vi "main.vi"() -> ()   [LabVIEW 2013]
doc: "Use this template to parse data you acquired from an instrument and write the data to a file.\nNote: LabVIEW enables automatic error handling by default for VIs you create from this template."
uses:
  Instance           1 22Saved   Instr_Read.vit .vi
  <vilib>/express/express shared/transition.llb/Dynamic To Waveform Array.vi
  <vilib>/Utility/file.llb/Write To Spreadsheet File (DBL).vi
  <vilib>/express/express signal manip/GetorSetDDTAttributes/Get DDT Attributes/Get DDT Properties.xnode
panel:
  out "Timestamp":timestamp
  in  "Pressão":dbl
  in  "Vazão":dbl
  out "P1 3":dbl(knob) scale=0.0..10.0
  out "P1 2":dbl(knob) scale=0.0..10.0
  out "P1":dbl(knob) scale=0.0..10.0 scale format="%#_2g"
  out "EMCA":cluster{dbl, dbl}(slide) scale=0.0..100.0 scale format="%#.2f %%"
  out "Água":dbl(slide) scale=0.0..100.0 scale format="%#.2f %%"
  out "ÁGUA\n              DE \nDESLOCAMENTO":dbl(slide) scale=0.0..100.0 scale format="%#.2f %%"
  in  "ON_OFF_Buttom":bool
  in  "Tab Control":enum32{"Entrada", "Aquisição", "Gráficos"}(tab)
  in  "Viscosidade (µ)":dbl=0.1
  in  "Comprimento (L)":dbl=4.0
  in  "Area (A)":dbl=2.0
  in  "Record_Buttom":bool
  in  "Arquivo de Aquisição":path
  in  "Taxa de Aquisição":dbl=1.0
  in  "Taxa de Atualização":dbl=10.0
  out "Waveform Graph 3":dynamicdata(graph)
  out "Waveform Graph 2":dynamicdata(graph)
  out "Waveform Graph 1":dynamicdata(graph)
  # "Bomba"
  # "Core Holder"
  # "On Windows/Linux, consider using the Instrument Driver Finder (Help>>Find Instrument Drivers) to search for an instrument driver for your instrument."
  # "m2"
  # "m"
  # "Pa.s"
  # "S/s"
  # "S/s"
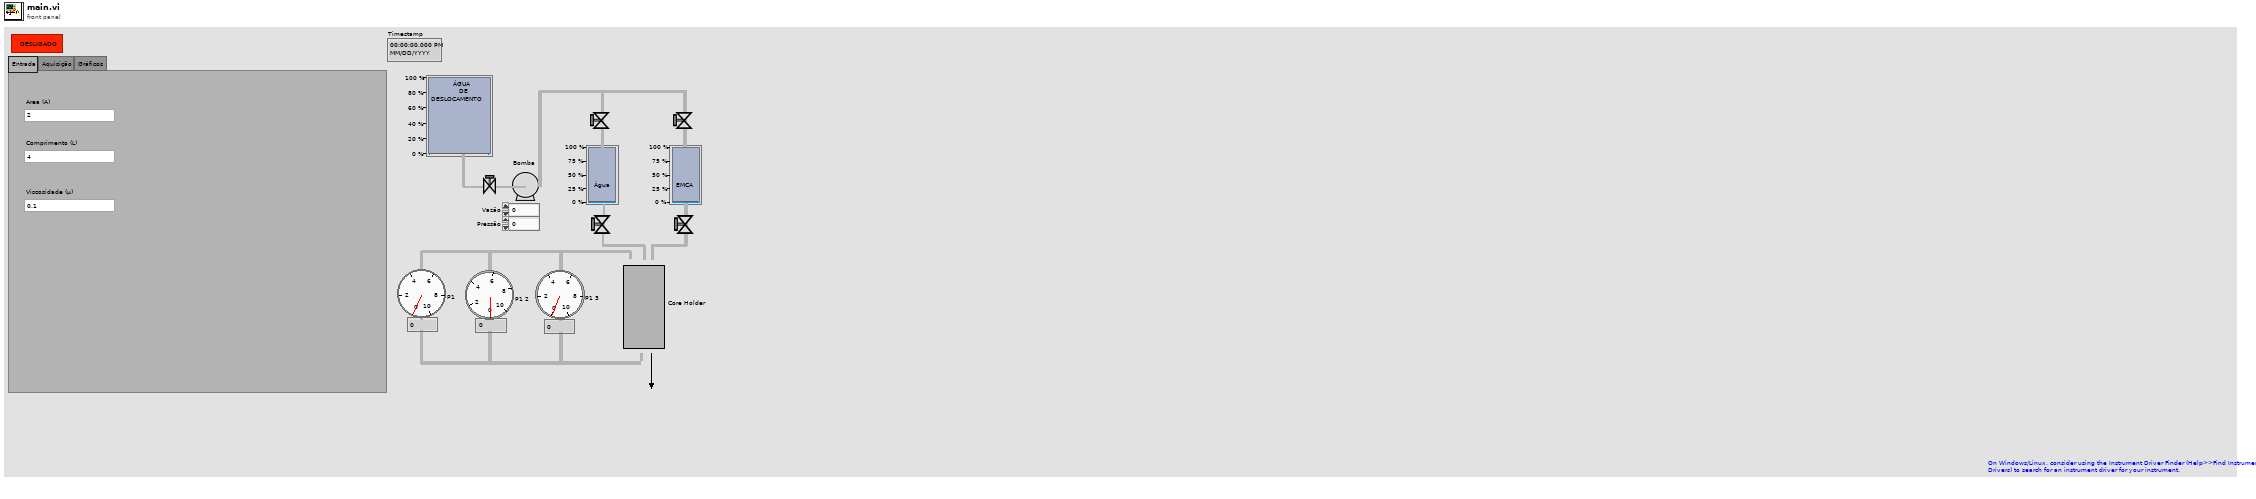
[diagram p1: front panel]
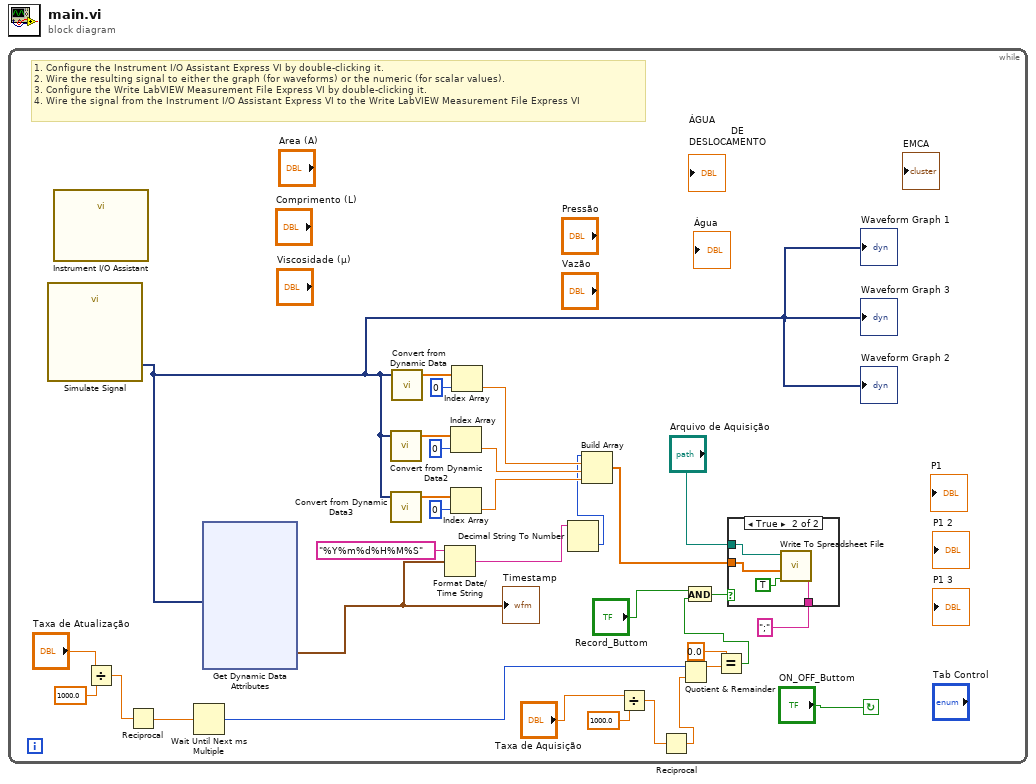
[diagram p0: block diagram]
diagram:
  n1 = while {
    stop <- "ON_OFF_Buttom" continue-if-true
    # "1. Configure the Instrument I/O Assistant Express VI by double-clicking it.\n2. Wire the resulting signal to either the graph (for waveforms) or the numeric (for scalar values).\n3. Configure the Write LabVIEW Measurement File Express VI by double-clicking it.\n4. Wire the signal from the Instrument I/O Assistant Express VI to the Write LabVIEW Measurement File Express VI"
    n2 = call "Simulate Signal"() -> ("Sine"=w9:dynamicdata)  [unwired: 14 in, 1 out]
    "Waveform Graph 3" <- w9
    "Waveform Graph 2" <- w9
    "Waveform Graph 1" <- w9
    n3 = call "Instrument I/O Assistant"() -> ()  [unwired: 12 in]
    n4 = Divide(x="Taxa de Atualização", y=1000.0) -> (x/y=w27:dbl)
    n5 = Reciprocal(x=w27) -> (1/x=w28:dbl)
    n6 = Wait Until Next ms Multiple(millisecond multiple=w28) -> (millisecond timer value=w29:u32)
    n7 = xnode "Get Dynamic Data Attributes"("Signals In"=w9) -> ("Timestamp"=w5:timestamp)  [unwired: 2 in, 3 out]
    "Timestamp" <- w5
    n8 = call "Convert from Dynamic Data2"("Dynamic Data Type"=w9) -> ("Array"=w13:dbl[])  [unwired: 3 in]
    n9 = call "Convert from Dynamic Data3"("Dynamic Data Type"=w9) -> ("Array"=w11:dbl[])  [unwired: 3 in]
    n10 = call "Convert from Dynamic Data"("Dynamic Data Type"=w9) -> ("Array"=w31:dbl[])  [unwired: 3 in]
    n11 = Format Date/Time String(time format string (%c)="%Y%m%d%H%M%S", seconds (now)=w5) -> (date/time string=w3:string)  [unwired: 1 in]
    n12 = Index Array(array=w13, index=0) -> (element=w7:dbl)
    n13 = Index Array(array=w11, index=0) -> (element=w6:dbl)
    n14 = Index Array(array=w31, index=0) -> (element=w8:dbl)
    n15 = Decimal String To Number(string=w3) -> (number=w2:i32)  [unwired: 2 in, 1 out]
    n16 = Build Array(w2, w8, w7, w6) -> (w1:dbl[])
    n17 = Divide(x="Taxa de Aquisição", y=1000.0) -> (x/y=w24:dbl)
    n18 = Reciprocal(x=w24) -> (1/x=w21:dbl)
    n19 = Quotient & Remainder(x=w29, y=w21) -> (x-y*floor(x/y)=w20:dbl)  [unwired: 1 out]
    n20 = Equal?(x=0.0, y=w20) -> (x = y?=w17:bool)
    n21 = And(x="Record_Buttom", y=w17) -> (x .and. y?=w16:bool)
    n22 = case shown="True" w16 {
      tunnel: "Arquivo de Aquisição" -> [_ w36]
      tunnel: ";" ("delimiter (\\t)") -> [_ w35]
      tunnel: w1 -> [_ w33]
      frame False {
      }
      frame True {
        n23 = call-poly <vilib>:"Write To Spreadsheet File.vi"("delimiter (\\t)"=w35, "append to file? (new file:F)"=TRUE, "1D data"=w33, "file path (dialog if empty)"=w36) -> ()  [unwired: 4 in, 1 out]
      }
    }
  }
